vi "Lua Load File.vi"(7 "mode (t)":string(combo)="t", 8 "error in (no error)":errorcluster, 10 "filename":path, 11 "Lua in":refnum<class "Lua.lvclass">) -> (0 "error out":errorcluster, 3 "Lua out":refnum<class "Lua.lvclass">)   [LabVIEW 2020, in "Lua for LabVIEW.lvlib" / "Lua.lvclass"]
doc: "Loads a lua file into the Lua state."
uses:
  Lua.lvclass
  Lua.lvclass/Lua.ctl
  lib/lua.dll/lua.dll.lvlib
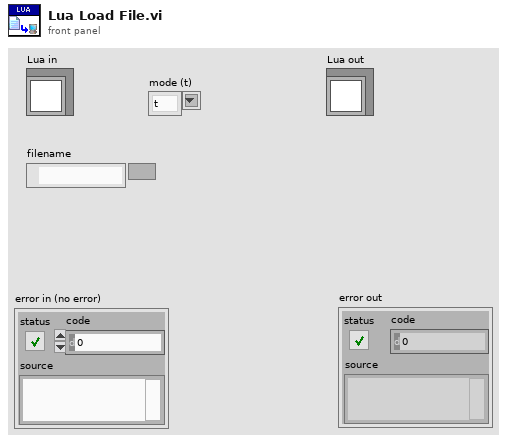
[diagram p1: front panel]
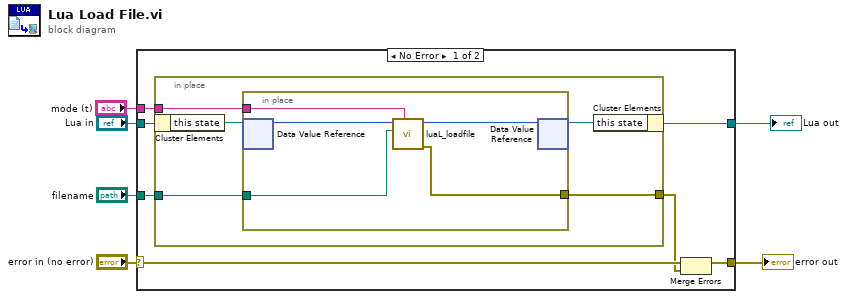
[diagram p0: block diagram]
diagram:
  n1 = case shown="No Error" "error in (no error)" {
    selector: "error in (no error)" -> [w13 w25]
    tunnel: [w10 w25] -> w5
    tunnel: "Lua in" -> [w12 w24]
    tunnel: [w8 w24] -> w3
    tunnel: "filename" -> [w11 _]
    tunnel: "mode (t)" -> [w7 _]
    frame No Error {
      n2 = in-place {
        in-place-border: w11 -> [w17]
        in-place-border: [w16] -> w9
        in-place-border: w7 -> [w14]
        n3 = in-place-cluster #1(w12) -> ("this state"=w18:refnum<data-value>)
        n4 = in-place {
          in-place-border: w17 -> [w22]
          in-place-border: [w21] -> w16
          in-place-border: w14 -> [w19]
          n5 = in-place-dvr #2(w18) -> (w23:u64)  [unwired: 1 out]
          n6 = call "luaL_loadfile.vi"("mode"=w19, "filename"=w22, "lua_state_p"=w23) -> ("error out"=w21:errorcluster, "lua_state_p out"=w20:u64)  [unwired: 7 in]
          n7 = in-place-dvr #2(w20) -> (w15:refnum<data-value>)  [unwired: 1 out]
        }
        n8 = in-place-cluster #1("this state"=w15) -> (w8:refnum<class "Lua.lvclass">)
      }
      n9 = Merge Errors(w13, w9) -> (w10:errorcluster)
    }
    frame Error {
    }
  }
  "Lua out" <- w3
  "error out" <- w5
